vi "选择规格.vi"(8 "error in (no error)":errorcluster caption="错误输入（无错误）", 9 "索引":i32, 10 "规格":refnum<class>[](array[class]), 11 "规格 输入":refnum<class "规格.lvclass">) -> (0 "error out":errorcluster caption="错误输出", 2 "特定类引用":refnum<class "规格.lvclass">, 3 "规格 输出":refnum<class "规格.lvclass">)   [LabVIEW 2016, in "规格.lvclass"]
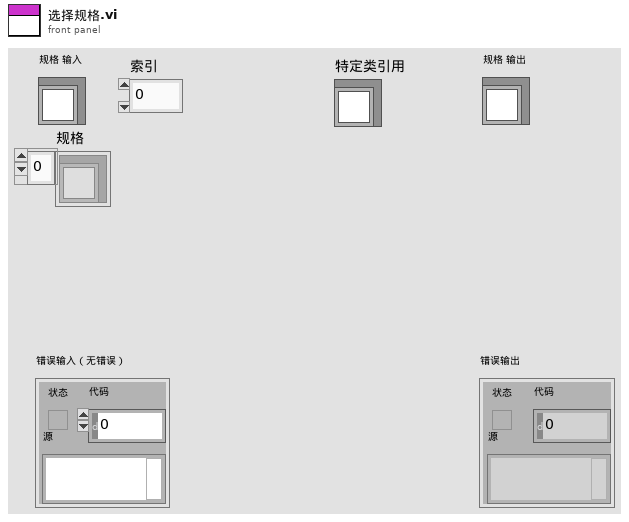
[diagram p1: front panel]
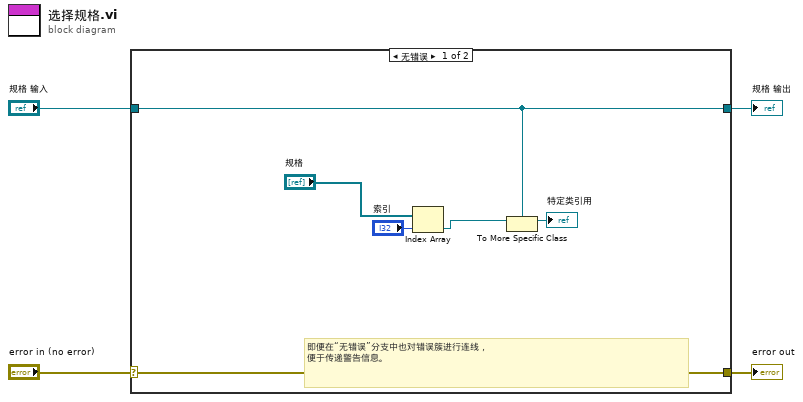
[diagram p0: block diagram]
diagram:
  n1 = case shown="无错误" "error in (no error)" {
    selector: "error in (no error)" -> [w10 w12]
    tunnel: [w10 w12] -> w3
    tunnel: [w8 w11] -> w1
    tunnel: "规格 输入" -> [w8 w11]
    frame No Error {
      # "即便在“无错误”分支中也对错误簇进行连线，\n便于传递警告信息。"
      n2 = Index Array(array="规格", index="索引") -> (element=w9:refnum<class>)
      n3 = To More Specific Class(target class=w8, reference=w9) -> (specific class reference=→"特定类引用":refnum<class "规格.lvclass">)  [unwired: 1 in, 1 out]
    }
    frame Error {
    }
  }
  "error out" <- w3
  "规格 输出" <- w1
